vi "TEST - Exotic Types.vi"(8 "error in (no error)":errorcluster) -> (0 "error out":errorcluster, 2 "pass":bool)   [LabVIEW 2020, in "test_openg_array.lvlib"]
uses:
  test_openg_array.lvlib
  source/library/openg_variant.lvlib
panel:
  in  "IMAQ Session":refnum<k11>
  in  "Waveform":waveform(dbl)={"t0"=timestamp(0 s since 1904-01-01), "dt"=0.0, "Y"=[]}
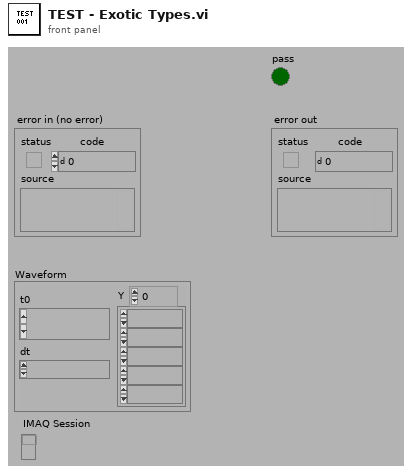
[diagram p1: front panel]
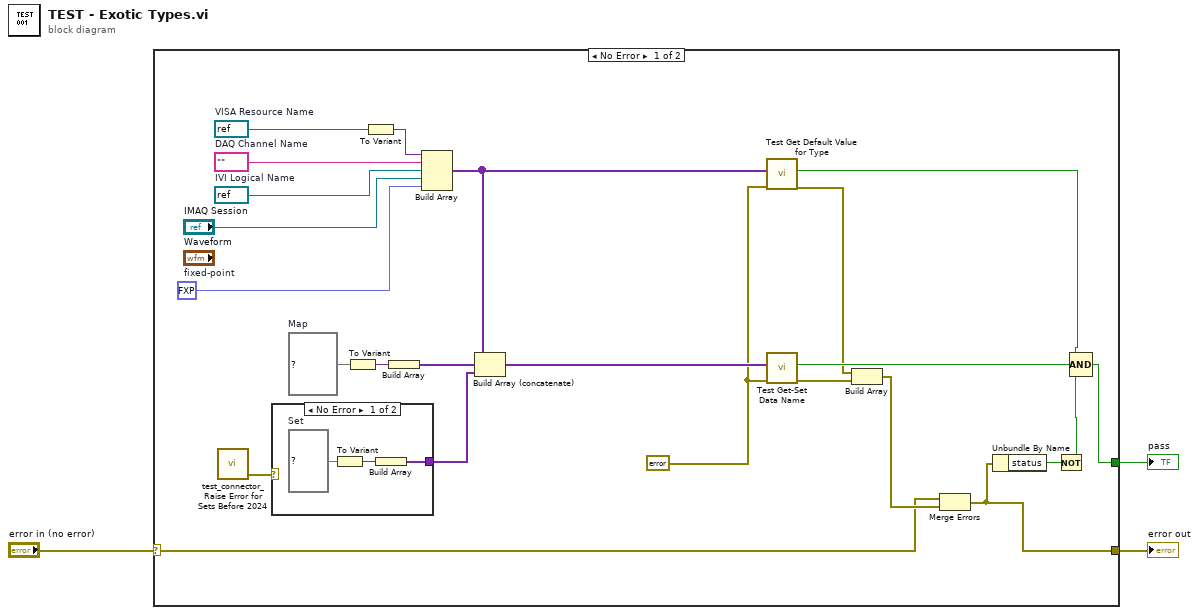
[diagram p0: block diagram]
diagram:
  n1 = case shown="No Error" "error in (no error)" {
    selector: "error in (no error)" -> [w5 w31]
    tunnel: [w17 _] -> w3
    tunnel: [w20 w31] -> w1
    frame No Error {
      w14 = map{string, i32} {}  # Map
      w21 = fxp<+/-,32,16> 0.0  # fixed-point
      w8 = errorcluster {"status"=FALSE, "code"=0, "source"=""} ("error out")
      w23 = refnum<k15> refnum  # IVI Logical Name
      w26 = refnum<visa-resource-name> refnum  # VISA Resource Name
      w24 = tag ""  # DAQ Channel Name
      n2 = call "test_connector_Raise Error for Sets Before 2024.vi"() -> ("error out"=w4:errorcluster)  [unwired: 10 in, 1 out]
      n3 = case shown="No Error" w4 {
        tunnel: [w30 _] -> w16
        frame No Error {
          w29 = set{string} {}  # Set
          n4 = To Variant(anything=w29) -> (Variant=w28:variant)
          n5 = Build Array(w28) -> (w30:variant[])
        }
        frame Error {
        }
      }
      n6 = To Variant(anything=w14) -> (Variant=w13:variant)
      n7 = To Variant(anything=w26) -> (Variant=w25:variant)
      n8 = Build Array(w13) -> (w15:variant[])
      n9 = Build Array(w25, w24, w23, "IMAQ Session", w21) -> (w6:variant[])
      n10 = Build Array (concatenate)(w6, w15, w16) -> (w12:variant[])
      n11 = call "Test Get Default Value for Type.vi"("error in"=w8, "types to test"=w6) -> ("error out"=w7:errorcluster, "passed"=w9:bool)  [unwired: 8 in]
      n12 = call "Test Get-Set Data Name.vi"("error in (no error)"=w8, "types to test"=w12) -> ("error out"=w11:errorcluster, "Passed"=w10:bool)  [unwired: 8 in]
      n13 = Build Array(w7, w11) -> (w27:errorcluster[])
      n14 = Merge Errors(w5, w27) -> (w20:errorcluster)
      n15 = Unbundle By Name(w20) -> ("status"=w19:bool)
      n16 = Not(x=w19) -> (.not. x?=w18:bool)
      n17 = Compound Arithmetic op=AND(w9, w10, w18) -> (w17:bool)
    }
    frame Error {
    }
  }
  "pass" <- w3
  "error out" <- w1
